vi "ControlPlotBalls.vi"(1 "Y-center":dbl(slide) scale=-10.0..10.0, 2 "x-center":dbl(slide) scale=-10.0..10.0) -> (0 "XY Graph":cluster{dbl[], dbl[]}(graph))   [LabVIEW 2014]
panel:
  in  "Color":u32(colorbox)
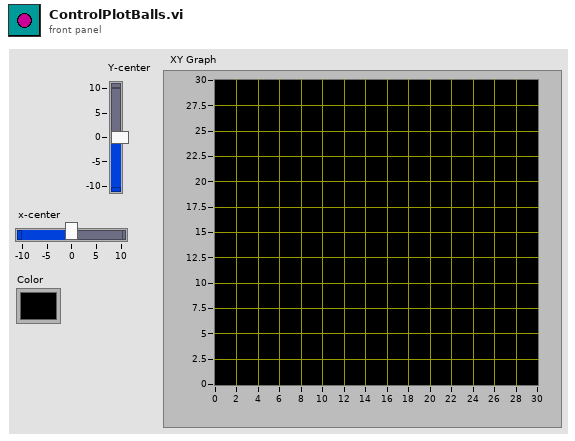
[diagram p1: front panel]
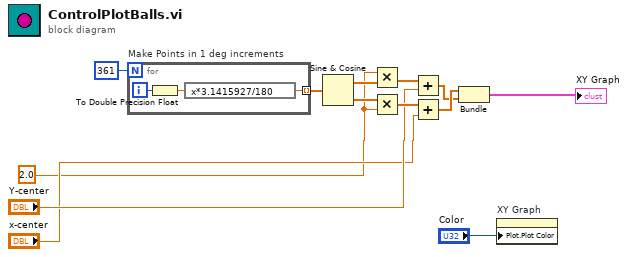
[diagram p0: block diagram]
diagram:
  w1 = 2.0
  n1 = for "Make Points in 1 deg increments" {
    N: 361 -> [_]
    tunnel: [w14] -> w6 mode=indexing
    i -> [w16]
    n2 = To Double Precision Float(number=w16) -> (double precision float=w15:dbl)
    n3 = expression code="x*3.1415927/180"(w15) -> (w14:dbl)
  }
  n4 = Sine & Cosine(0:w6) -> (1:w7:dbl[], 2:w8:dbl[])
  n5 = Multiply(x=w1, y=w7) -> (x*y=w10:dbl[])
  n6 = Multiply(x=w8, y=w1) -> (x*y=w12:dbl[])
  n7 = Add(x=w10, y="Y-center") -> (x+y=w11:dbl[])
  n8 = Add(x=w12, y="x-center") -> (x+y=w13:dbl[])
  n9 = Bundle(w13, w11) -> (→"XY Graph":cluster{dbl[], dbl[]})  [unwired: 1 in]
  n10 = property on="XY Graph" class="XYGraph (strict)"("Plot.Plot Color"="Color") -> ()  [unwired: 2 in, 2 out]
